vi "VescTestVISA.vi"() -> ()   [LabVIEW 2019]
uses:
  <vilib>/myRIO/Instrument Drivers/Onboard IO/UART/typedef/VISA Configuration.ctl
  <vilib>/Instr/_visa.llb/VISA Configure Serial Port (Instr).vi
  <vilib>/myRIO/Express VI/Onboard IO/UART/UART Express VI.xnode
  <vilib>/myRIO/Instrument Drivers/Onboard IO/UART/UART.lvlib
  usr/local/lib/libcrc16.so
panel:
  in  "RPM":u32
  out "return count":u32
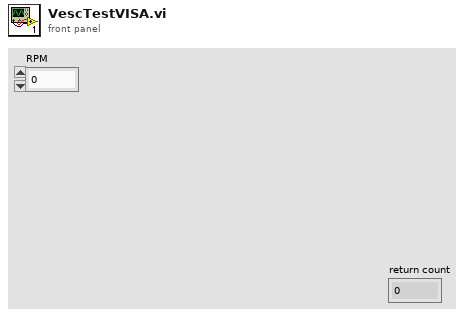
[diagram p1: front panel]
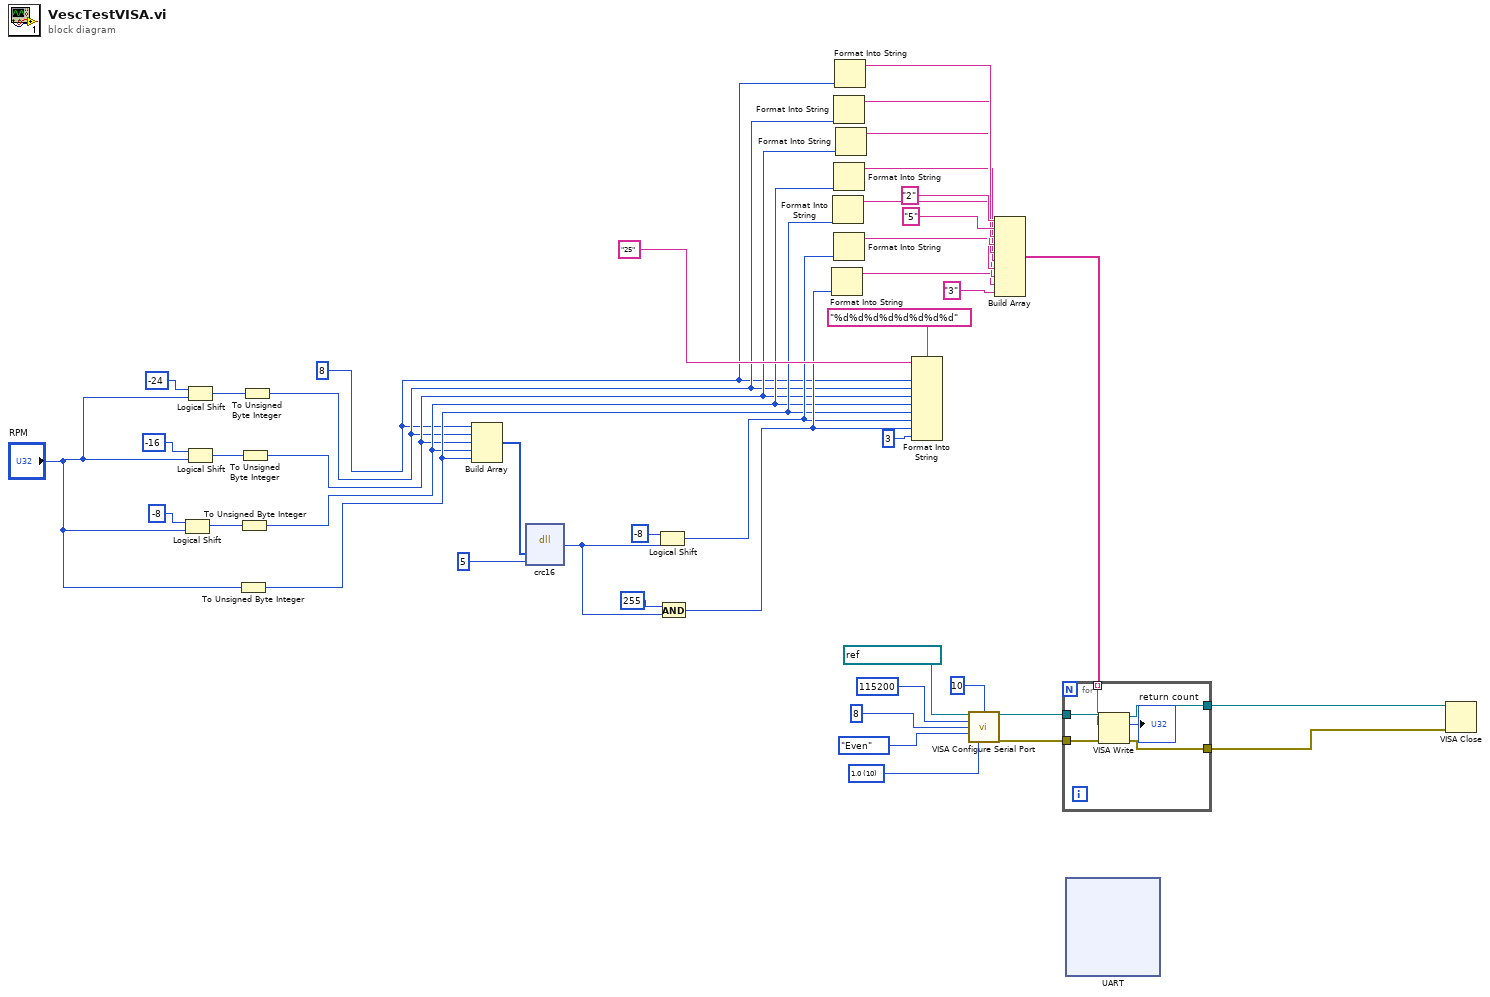
[diagram p0: block diagram]
diagram:
  w9 = 8
  w39 = u16 10 items=["1.0"=10, "1.5"=15, "2.0"=20] ("stop bits (10: 1 bit)")
  n1 = Logical Shift(y=i16 -8, x="RPM") -> (x << y=w28:u32)
  n2 = Logical Shift(y=i16 -24, x="RPM") -> (x << y=w32:u32)
  n3 = Logical Shift(y=i16 -16, x="RPM") -> (x << y=w29:u32)
  n4 = To Unsigned Byte Integer(number="RPM") -> (unsigned 8bit integer=w13:u8)
  n5 = To Unsigned Byte Integer(number=w28) -> (unsigned 8bit integer=w12:u8)
  n6 = To Unsigned Byte Integer(number=w29) -> (unsigned 8bit integer=w11:u8)
  n7 = To Unsigned Byte Integer(number=w32) -> (unsigned 8bit integer=w10:u8)
  n8 = Build Array(w9, w10, w11, w12, w13) -> (w26:i32[])
  n9 = dll-call lib="usr/local/lib/libcrc16.so" fn="crc16"("buf"=w26, "len"=5) -> ("return type"=w21:u8)  [unwired: 5 in, 2 out]
  n10 = Logical Shift(y=i16 -8, x=w21) -> (x << y=w14:u8)
  n11 = And(x=u8 255, y=w21) -> (x .and. y?=w15:u8)
  n12 = Format Into String(w15) -> (resulting string=w2:string)  [unwired: 3 in, 1 out]
  n13 = Format Into String(w13) -> (resulting string=w4:string)  [unwired: 3 in, 1 out]
  n14 = Format Into String(w10) -> (resulting string=w7:string)  [unwired: 3 in, 1 out]
  n15 = Format Into String(w12) -> (resulting string=w5:string)  [unwired: 3 in, 1 out]
  n16 = Format Into String(w14) -> (resulting string=w3:string)  [unwired: 3 in, 1 out]
  n17 = Format Into String(w9) -> (resulting string=w8:string)  [unwired: 3 in, 1 out]
  n18 = Format Into String(w11) -> (resulting string=w6:string)  [unwired: 3 in, 1 out]
  n19 = Format Into String(format string="%d%d%d%d%d%d%d%d", initial string="25", w9, w10, w11, w12, w13, w14, w15, u8 3 ("input 8")) -> ()  [unwired: 1 in, 2 out]
  n20 = call-poly "VISA Configure Serial Port"("VISA resource name"=refnum<visa-resource-name> "ASRL2::INSTR", "termination char\n(0xA = '\\n' = LF)"=u8 10 ("termination char\n(0xA = '\\n' = LF)"), "baud rate (9600)"=u32 115200, "data bits (8)"=u16 8, "parity (0:none)"=enum16{"None", "Odd", "Even", "Mark", "Space"}."Even", "stop bits (10: 1 bit)"=w39) -> ("VISA resource name out"=w37:refnum<visa-resource-name>, "error out"=w34:errorcluster)  [unwired: 8 in]
  n21 = Build Array("2", "5", w8, w7, w6, w5, w4, w3, w2, "3") -> (w1:string[])
  n22 = for {
    tunnel: w37 -> [w49]
    tunnel: [w48] -> w36
    tunnel: [w46] -> w35
    tunnel: w34 -> [w45]
    tunnel: w1 -> [w44] mode=indexing
    n23 = VISA Write(VISA resource name=w49, write buffer=w44, error in (no error)=w45) -> (VISA resource name out=w48:refnum<visa-resource-name>, return count=→"return count":u32, error out=w46:errorcluster)
  }
  n24 = xnode "UART"() -> ()  [unwired: 2 in, 2 out]
  n25 = VISA Close(VISA resource name=w36, error in (no error)=w35) -> ()  [unwired: 1 out]
